vi "Run_VI.vi"(8 "error in (no error)":errorcluster, 9 "Message_command_in":T1, 10 "Command Queue in":T2) -> (0 "error out":errorcluster, 1 "Message_command out":T1, 2 "Command Queue out":T2, 11 "machine name (\"\":  open local reference)":string)   [LabVIEW 2019]
uses:
  Command_Queue.ctl
  Command_Message.ctl
panel:
  out "error out 2":errorcluster
  in  "port":u16=3374
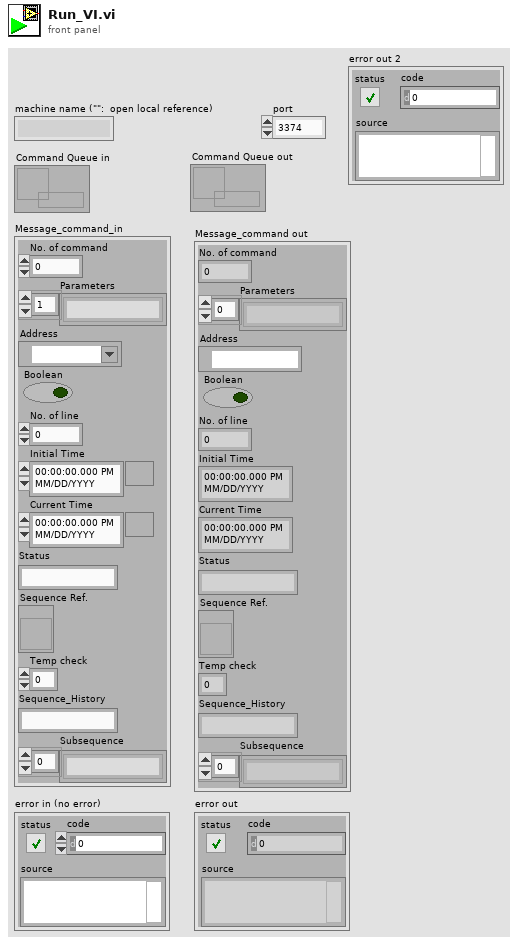
[diagram p1: front panel]
types:
  T1 = typedef "Command_Message.ctl" = cluster{"No. of command":i32, "Parameters":string[], "Address":refnum<visa-resource-name>, "Boolean":bool, "No. of line":i32, "Initial Time":timestamp, "Current Time":timestamp, "Status":string, "Sequence Ref.":refnum<vi>, "Temp check":i32, "Sequence_History":string, "Subsequence":string[]}
  T2 = typedef "Command_Queue.ctl" = refnum<queue>
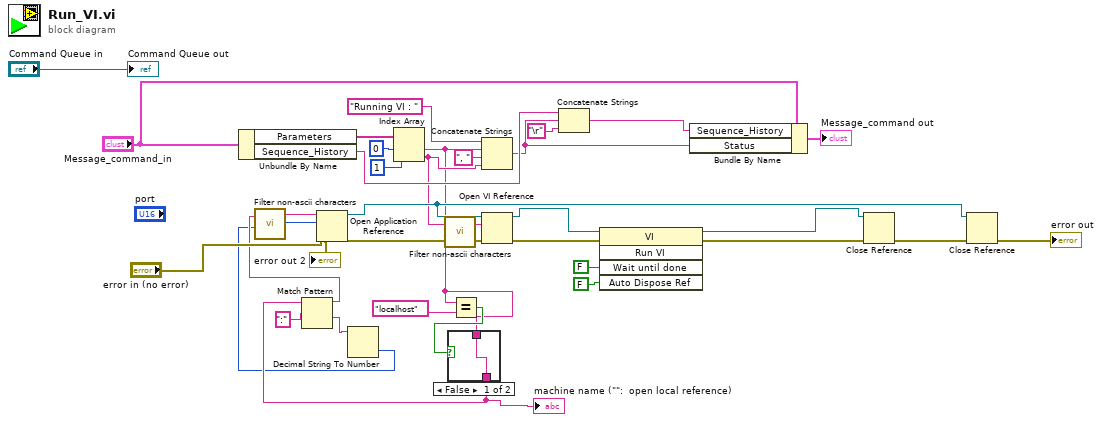
[diagram p0: block diagram]
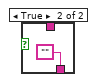
[diagram p2: hidden frame]
diagram:
  n1 = Unbundle By Name("Message_command_in") -> ("Parameters"=w33:string[], "Sequence_History"=w23:string)
  n2 = Index Array(array=w33, index #1=0 ("index"), index #2=1 ("index")) -> (element #1=w13:string, element #2=w17:string)
  n3 = call "Filter non-ascii characters.vi"(2:w17) -> ("output"=w6:string)  [unwired: 1 in]
  n4 = Equal?(x=w13, y="localhost") -> (x = y?=w14:bool)
  n5 = case shown="False" w14 {
    tunnel: [w35 ""] -> w12
    tunnel: w13 -> [w35 _]
    frame False {
    }
    frame True {
    }
  }
  "machine name (\"\":  open local reference)" <- w12
  n6 = Match Pattern(string=w12, regular expression=":") -> (before substring=w10:string, after substring=w9:string)  [unwired: 1 in, 2 out]
  n7 = call "Filter non-ascii characters.vi"(2:w10) -> ("output"=w7:string)  [unwired: 1 in]
  n8 = Decimal String To Number(string=w9) -> (number=w8:i32)  [unwired: 2 in, 1 out]
  n9 = Open Application Reference(8:"error in (no error)", 10:w8, 11:w7) -> (0:w5:errorcluster, 3:w26:refnum<vi>)  [unwired: 1 in]
  "error out 2" <- w5
  n10 = Concatenate Strings("Running VI : " ("string"), w13, ", " ("string"), w17) -> (w20:string)
  n11 = Open VI Reference(application reference (local)=w26, vi path=w6, error in (no error)=w5) -> (vi reference=w30:refnum<vi>, error out=w4:errorcluster)  [unwired: 3 in]
  n12 = Concatenate Strings(w23, w20, "\r") -> (w21:string)
  n13 = invoke class="VI" method="Run VI"(reference=w30, error in=w4, "Wait until done"=FALSE ("Wait Until Done"), "Auto Dispose Ref"=FALSE ("Auto Dispose Reference")) -> (reference out=w27:refnum<vi>, error out=w3:errorcluster)  [unwired: 1 in, 3 out]
  n14 = Bundle By Name(cluster="Message_command_in", "Sequence_History"=w21, "Status"=w20) -> (→"Message_command out":T1)
  n15 = Close Reference(reference=w27, error in (no error)=w3) -> (error out=w2:errorcluster)
  n16 = Close Reference(reference=w26, error in (no error)=w2) -> (error out=→"error out":errorcluster)
  "Command Queue out" <- "Command Queue in"
